vi "Cents2DollarString.vi"() -> ()   [LabVIEW 2019]
panel:
  out "Dollars":string
  in  "Cents":dbl
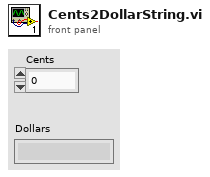
[diagram p1: front panel]
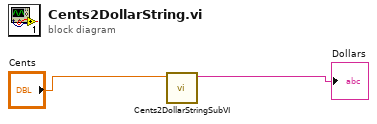
[diagram p0: block diagram]
diagram:
  n1 = call "Cents2DollarStringSubVI.vi"("Cents"="Cents") -> ("String"=→"Dollars":string)  [unwired: 10 in]
